vi "simulate_Measurement.vi"(8 "error in (no error)":errorcluster, 10 "Function in":T1, 11 "Measurement in":T3 {"Channel Status" format="%02x"}) -> (0 "error out":errorcluster, 2 "Function out":T1, 3 "Measurement out":T3 {"Channel Status" format="%02x"})   [LabVIEW 2019, in "SimELoad.lvlib" / "SimEload.lvclass"]
uses:
  SimEload.lvclass
  builds/Instruments/Electronic Load.lvlibp/Custom Controls/Measured Values.ctl
  builds/Instruments/Electronic Load.lvlibp/Custom Controls/E-Load Function.ctl
  builds/Instruments/Electronic Load.lvlibp/Custom Controls/E-Load Mode.ctl
  builds/Instruments/Electronic Load.lvlibp/Electronic Load.lvclass
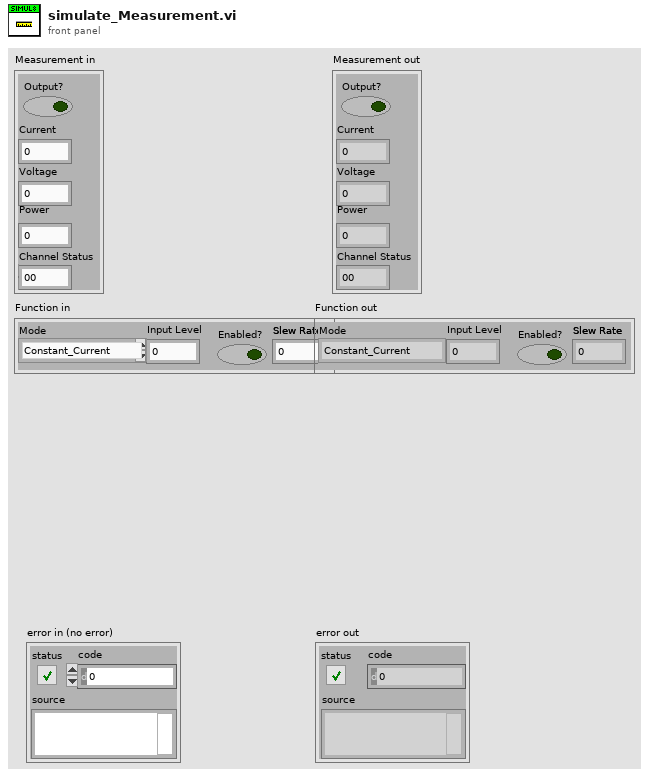
[diagram p1: front panel]
types:
  T1 = typedef "Electronic Load.lvlibp/Electronic Load.lvclass/E-Load Function.ctl" = cluster{"Mode":T2, "Input Level":dbl, "Enabled?":bool, "Slew Rate":dbl}
  T2 = typedef "Electronic Load.lvlibp/Electronic Load.lvclass/E-Load Mode.ctl" = enum16{"Constant_Current", "Constant_Resistance", "Constant_Voltage"}
  T3 = typedef "Electronic Load.lvlibp/Electronic Load.lvclass/Measured Values.ctl" = cluster{"Output?":bool, "Current":dbl, "Voltage":dbl, "Power":dbl, "Channel Status":i32}
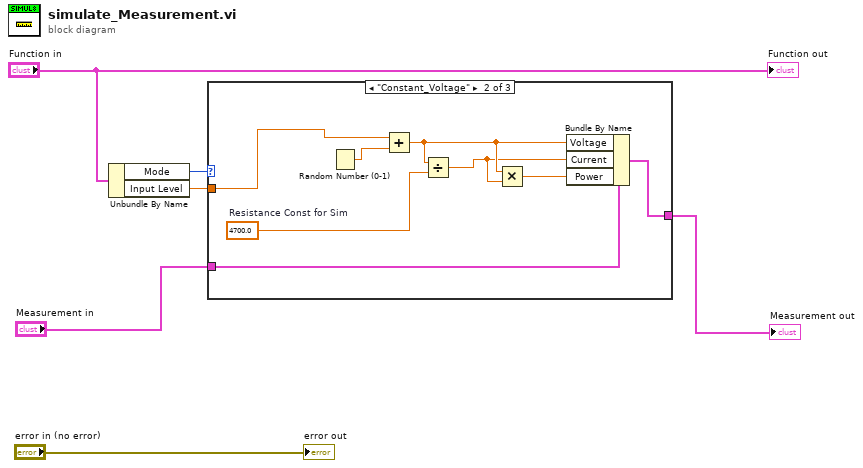
[diagram p0: block diagram]
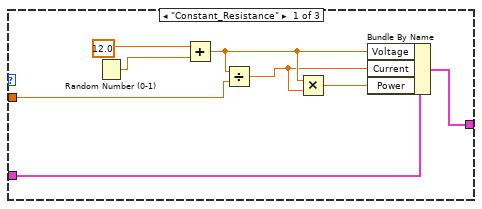
[diagram p2: hidden frame]
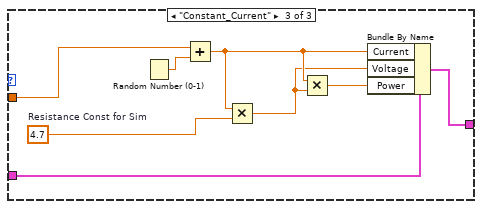
[diagram p3: hidden frame]
diagram:
  n1 = Unbundle By Name("Function in") -> ("Mode"=w5:T2, "Input Level"=w4:dbl)
  n2 = case shown="\"Constant_Voltage\"" w5 {
    tunnel: w4 -> [w8 w15 w23]
    tunnel: "Measurement in" -> [w14 w22 w30]
    tunnel: [w13 w21 w29] -> w2
    frame "Constant_Resistance" {
      n3 = Random Number (0-1)() -> (number: 0 to 1=w9:dbl)
      n4 = Add(x=12.0, y=w9) -> (x+y=w12:dbl)
      n5 = Divide(x=w12, y=w8) -> (x/y=w11:dbl)
      n6 = Multiply(x=w12, y=w11) -> (x*y=w10:dbl)
      n7 = Bundle By Name(cluster=w14, "Voltage"=w12, "Current"=w11, "Power"=w10) -> (w13:T3)
    }
    frame "Constant_Voltage" {
      w17 = 4700.0  # Resistance Const for Sim
      n8 = Random Number (0-1)() -> (number: 0 to 1=w16:dbl)
      n9 = Add(x=w15, y=w16) -> (x+y=w20:dbl)
      n10 = Divide(x=w20, y=w17) -> (x/y=w19:dbl)
      n11 = Multiply(x=w20, y=w19) -> (x*y=w18:dbl)
      n12 = Bundle By Name(cluster=w22, "Voltage"=w20, "Current"=w19, "Power"=w18) -> (w21:T3)
    }
    frame "Constant_Current" {
      w28 = 4.7  # Resistance Const for Sim
      n13 = Random Number (0-1)() -> (number: 0 to 1=w24:dbl)
      n14 = Add(x=w23, y=w24) -> (x+y=w27:dbl)
      n15 = Multiply(x=w27, y=w28) -> (x*y=w26:dbl)
      n16 = Multiply(x=w27, y=w26) -> (x*y=w25:dbl)
      n17 = Bundle By Name(cluster=w30, "Current"=w27, "Voltage"=w26, "Power"=w25) -> (w29:T3)
    }
  }
  "Measurement out" <- w2
  "Function out" <- "Function in"
  "error out" <- "error in (no error)"
